vi "Read Data.vi"(8 "error in (no error)":errorcluster, 11 "LakeShore370 in":refnum<class "LakeShore370_device.lvclass">) -> (0 "error out":errorcluster, 2 "Data":waveform(dbl)[](array[waveform]), 3 "LakeShore370 out":refnum<class "LakeShore370_device.lvclass">)   [LabVIEW 2015, in "LakeShore370_device.lvclass"]
uses:
  LakeShore370_device.lvclass
  LakeSore370 Front Panel Data.ctl
  LakeShore370 Heater Ranges.ctl
  Neocera/Neocera Set Point Aproach.ctl
  OO Devices/Device/Read Controls Snapshot.vi
  Instrument/Read VISA Resource.vi
  OO Devices/Device/Read Control Panel Loaded.vi
  Get LakeShore 370 Resistance_VISA.vi
  Instrument/Write VISA Resource.vi
  Instrument with scanner/Instrument with scanner.lvclass
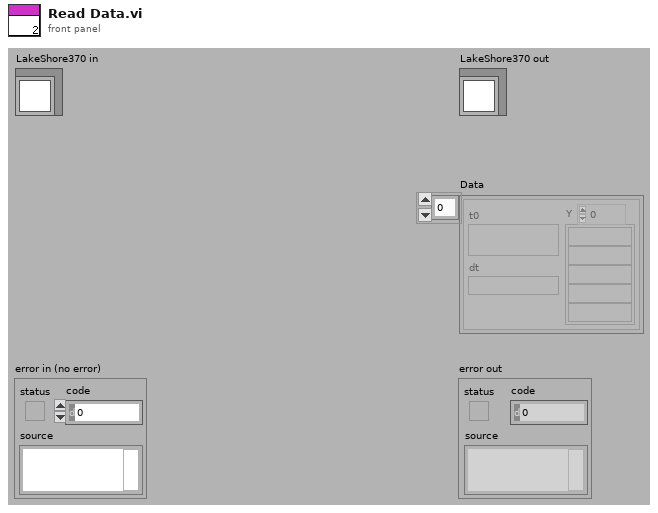
[diagram p1: front panel]
types:
  T1 = typedef "LakeSore370 Front Panel Data.ctl" = cluster{"Channels to scan":i32[], "Scan settling, s":dbl, "Read temperature":bool, "Set point":dbl, "Heater range":T2, "Approach":T3, "Ramp rate, K/min":dbl, "Read heater":bool}
  T2 = typedef "LakeShore370 Heater Ranges.ctl" = enum16{"Off", "31.6uA", "100uA", "316uA", "1mA", "3.16uA", "10mA", "31.6mA", "100mA"}
  T3 = typedef "Neocera Set Point Aproach.ctl" = enum16{"Instant", "Ramp"}
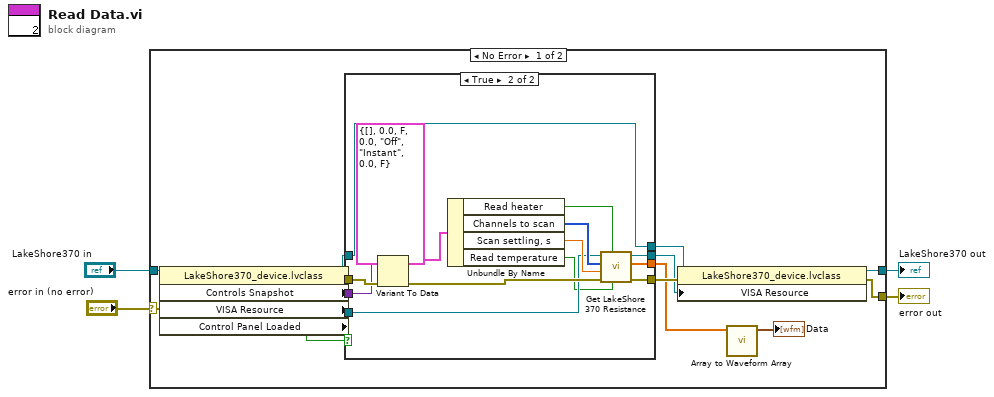
[diagram p0: block diagram]
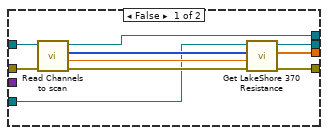
[diagram p2: hidden frame]
diagram:
  n1 = case shown="No Error" "error in (no error)" {
    selector: "error in (no error)" -> [w16 w44]
    tunnel: [w14 w44] -> w3
    tunnel: [w15 w43] -> w1
    tunnel: "LakeShore370 in" -> [w18 w43]
    frame No Error {
      n2 = property class="LakeShore370_device.lvclass"(reference=w18, error in=w16) -> (reference out=w17:refnum<class "LakeShore370_device.lvclass">, error out=w11:errorcluster, "Controls Snapshot"=w5:variant, "VISA Resource"=w8:refnum<visa-resource-name>, "Control Panel Loaded"=w6:bool)
      n3 = case shown="True" w6 {
        tunnel: w17 -> [w28 w35]
        tunnel: [w27 w35] -> w13
        tunnel: [w26 w36] -> w12
        tunnel: w11 -> [w24 w40]
        tunnel: [w19 w34] -> w9
        tunnel: w8 -> [w21 w33]
        tunnel: [w20 w32] -> w7
        tunnel: w5 -> [_ w31]
        frame False {
          n4 = call "Read Channels to scan.vi"("error in (no error)"=w24, "Instrument with scanner.lvclass in"=w28) -> ("error out"=w25:errorcluster, "Seconds between samples"=w22:dbl, "Channels to scan (empty - don't use scanner option)"=w23:i32[], "Instrument with scanner.lvclass out"=w27:refnum<class "LakeShore370_device.lvclass">)  [unwired: 6 out]
          n5 = call-poly "Get LakeShore 370 Resistance.vi"("error in (no error)"=w25, "Seconds between samples"=w22, "Channels to scan (empty = don't use scanner option)"=w23, "VISA resource name"=w21) -> ("error out"=w26:errorcluster, "Resistance"=w19:dbl[], "VISA resource name out"=w20:refnum<visa-resource-name>)  [unwired: 2 in, 3 out]
        }
        frame True {
          n6 = Variant To Data(error in=w40, type=T1 {"Channels to scan"=[], "Scan settling, s"=0.0, "Read temperature"=FALSE, "Set point"=0.0, "Heater range"=enum."Off", "Approach"=enum."Instant", "Ramp rate, K/min"=0.0, "Read heater"=FALSE} ("Data"), Variant=w31) -> (data=w41:T1, error out=w39:errorcluster)
          n7 = Unbundle By Name(w41) -> ("Read heater"=w29:bool, "Channels to scan"=w38:i32[], "Scan settling, s"=w37:dbl, "Read temperature"=w30:bool)
          n8 = call-poly "Get LakeShore 370 Resistance.vi"("Read temperature"=w30, "Read heater"=w29, "error in (no error)"=w39, "Seconds between samples"=w37, "Channels to scan (empty = don't use scanner option)"=w38, "VISA resource name"=w33) -> ("error out"=w36:errorcluster, "Resistance"=w34:dbl[], "VISA resource name out"=w32:refnum<visa-resource-name>)  [unwired: 3 out]
        }
      }
      n9 = property class="LakeShore370_device.lvclass"(reference=w13, error in=w12, "VISA Resource"=w7) -> (reference out=w15:refnum<class "LakeShore370_device.lvclass">, error out=w14:errorcluster)
      n10 = call "Array to Waveform Array.vi"("Array"=w9) -> ("Waveform"=→"Data":waveform(dbl)[])  [unwired: 10 in]
    }
    frame Error {
    }
  }
  "error out" <- w3
  "LakeShore370 out" <- w1
